vi "Write Tenable.vi"(8 "error in (no error)":errorcluster, 10 "Tenable":refnum<k21>="PAS_TEC_En", 11 "ePAS in":refnum<class "ePAS.lvclass">) -> (0 "error out":errorcluster, 3 "ePAS out":refnum<class "ePAS.lvclass">)   [LabVIEW 2014, in "ePAS.lvclass"]
uses:
  ePAS.lvclass
  ePAS.lvclass/ePAS.ctl
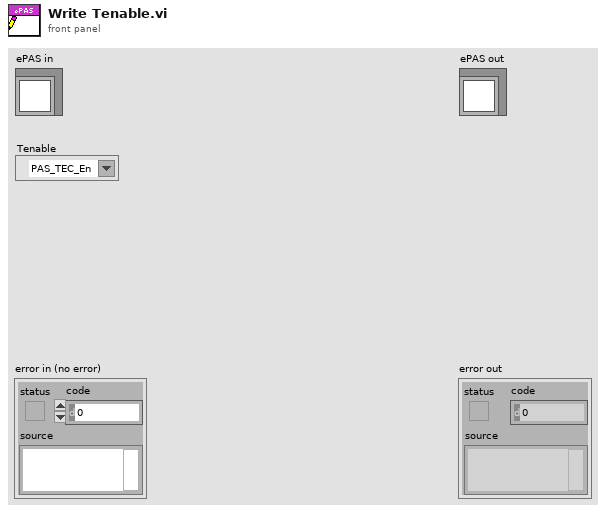
[diagram p1: front panel]
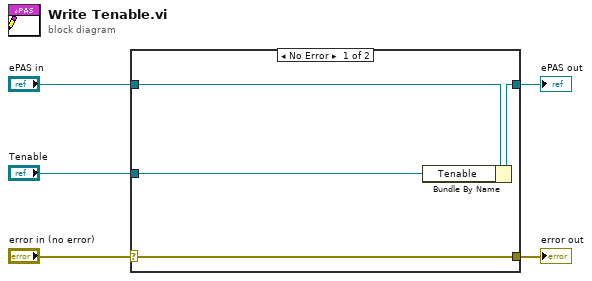
[diagram p0: block diagram]
diagram:
  n1 = case shown="No Error" "error in (no error)" {
    selector: "error in (no error)" -> [w9 w10]
    tunnel: [w9 w10] -> w4
    tunnel: [w7 w11] -> w2
    tunnel: "ePAS in" -> [w8 w11]
    tunnel: "Tenable" -> [w6 _]
    frame No Error {
      n2 = Bundle By Name(cluster=w8, "Tenable"=w6) -> (w7:refnum<class "ePAS.lvclass">)
    }
    frame Error {
    }
  }
  "error out" <- w4
  "ePAS out" <- w2
